vi "Tcheck.vi"(0 "TargetT":dbl, 1 "timeout (s)":dbl=600.0, 2 "Direct reading":bool, 3 "VI name":string="Tmonitor.vi", 5 "target T\nDT error":dbl=0.001 format="%#_13g", 7 "VISA resource name":refnum<visa-resource-name>, 9 "T to watch":string="T0", 11 "T control mode":u16(ring) items=["Tprobe", "Tsorb", "Fast Tsweep", "Skip T stable"], 14 "Pass":bool) -> (4 "Temp OK":bool, 6 "Temp close to\nTarget T":bool, 10 "time passed (s)":dbl=37.23 format="%#_4g", 15 "Temp":dbl=155.435 format="%#_4g")   [LabVIEW 2025]
uses:
  <vilib>/Analysis/baseanly.llb/Mean (DBL).vi
  <vilib>/Analysis/NI_AALBase.lvlib
panel:
  in  "Controller":u16(ring) items=["LS370", "LS340", "LS336"]
  in  "Channel":u16(ring) items=["A", "B", "C", "D", "4"]
  out "meanT":dbl format="%0.2f"
  out "min T":dbl
  out "max T":dbl
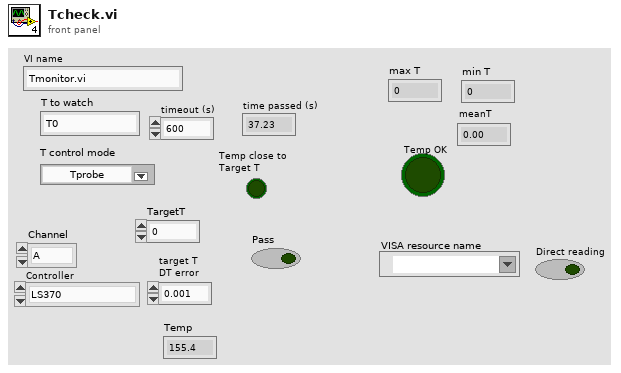
[diagram p1: front panel]
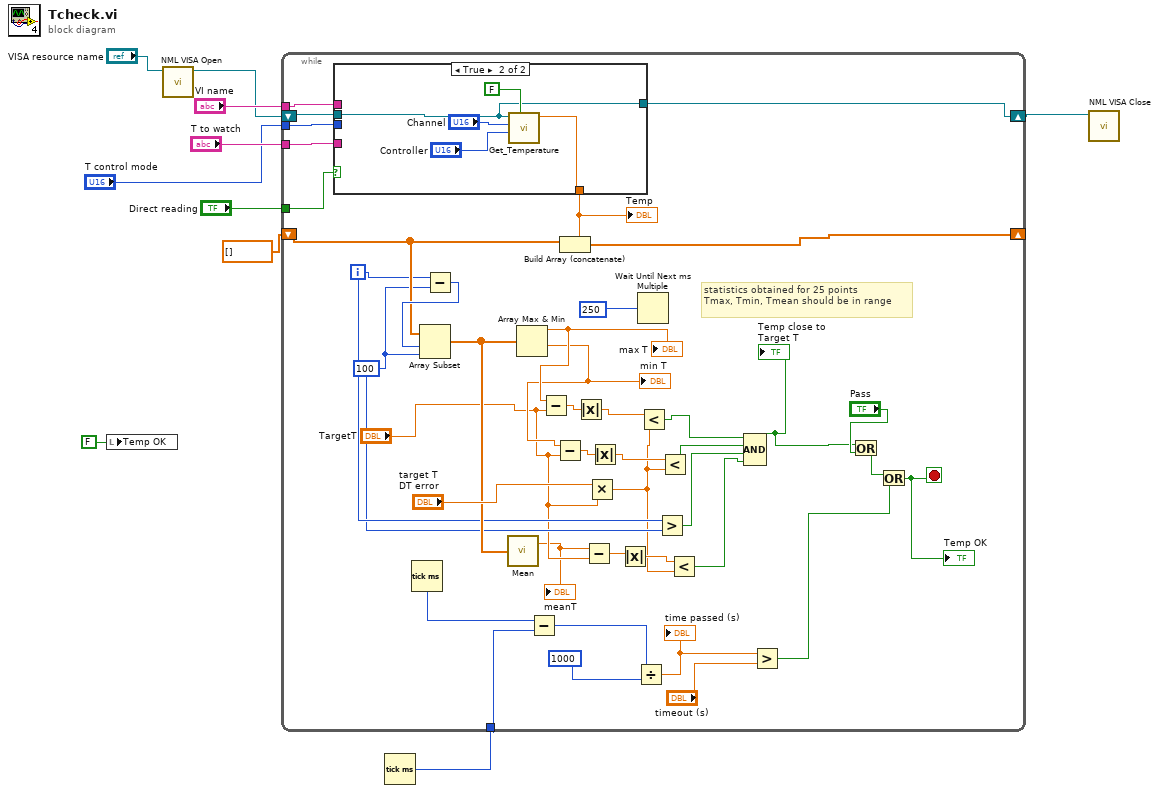
[diagram p0: block diagram]
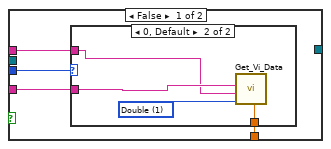
[diagram p2: hidden frame]
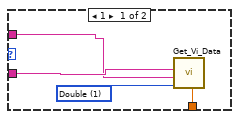
[diagram p3: hidden frame]
diagram:
  n1 = local write "Temp OK"(FALSE ("Temp OK")) -> ()
  n2 = call "NML VISA Open.vi"("VISA resource name"="VISA resource name") -> ("VISA resource name out"=w2:refnum<visa-resource-name>)  [unwired: 9 in, 1 out]
  n3 = Tick Count (ms)() -> (millisecond timer value=w10:u32)
  n4 = while {
    tunnel: w10 -> [w40]
    shift-right: [w37] -> _
    shift-left: dbl[] [] -> [w35]
    tunnel: "T to watch" -> [w17]
    tunnel: "T control mode" -> [w16]
    tunnel: "VI name" -> [w15]
    tunnel: "Direct reading" -> [w13]
    shift-right: [w11] -> w1
    shift-left: w2 -> [w12]
    i -> [w29]
    stop <- w14 stop-if-true
    w28 = 100 ("length")
    # "statistics obtained for 25 points\nTmax, Tmin, Tmean should be in range"
    n5 = case shown="True" w13 {
      tunnel: [w55 w65] -> w38
      tunnel: w17 -> [w54 _]
      tunnel: w16 -> [w53 _]
      tunnel: w15 -> [w52 _]
      tunnel: w12 -> [_ w64]
      tunnel: [_ w64] -> w11
      frame False {
        n6 = case shown="0, Default" w53 {
          tunnel: [w58 w62] -> w55
          tunnel: w54 -> [w57 w61]
          tunnel: w52 -> [w56 w60]
          frame 1 {
            w59 = u16 1 items=["String", "Double", "Boolean", "Variant"] ("Data Type")
            n7 = call "Get_Vi_Data.vi"("Data Type"=w59, "VI name"=w56, "Control Name"=w57) -> ("Data (Double)"=w58:dbl)  [unwired: 4 in, 4 out]
          }
          frame 0, Default {
            w63 = u16 1 items=["String", "Double", "Boolean", "Variant"] ("Data Type")
            n8 = call "Get_Vi_Data.vi"("Data Type"=w63, "VI name"=w60, "Control Name"=w61) -> ("Data (Double)"=w62:dbl)  [unwired: 4 in, 4 out]
          }
        }
      }
      frame True {
        n9 = call "Get_Temperature.vi"("Res?"=FALSE, "Controller"="Controller", "Channel"="Channel", "VISA resource name"=w64) -> ("Temperature"=w65:dbl)  [unwired: 6 in, 1 out]
      }
    }
    "Temp" <- w38
    n10 = Tick Count (ms)() -> (millisecond timer value=w47:u32)
    n11 = Subtract(x=w29, y=w28) -> (x-y=w36:i32)
    n12 = Array Subset(array=w35, index=w36, length=w28) -> (w30:dbl[])
    n13 = call-poly <vilib>:"Mean.vi"("X"=w30) -> ("mean"=w23:dbl)  [unwired: 1 out]
    "meanT" <- w23
    n14 = Array Max & Min(array=w30) -> (max value=w34:dbl, min value=w31:dbl)  [unwired: 2 out]
    "max T" <- w34
    "min T" <- w31
    n15 = Subtract(x=w47, y=w40) -> (x-y=w46:u32)
    n16 = Subtract(x=w34, y="TargetT") -> (x-y=w49:dbl)
    n17 = Subtract(x=w31, y="TargetT") -> (x-y=w32:dbl)
    n18 = Build Array (concatenate)(w35, w38) -> (w37:dbl[])
    n19 = Absolute Value(x=w49) -> (abs(x)=w50:dbl)
    n20 = Subtract(x=w23, y="TargetT") -> (x-y=w21:dbl)
    n21 = Multiply(x="target T\nDT error", y="TargetT") -> (x*y=w20:dbl)
    n22 = Absolute Value(x=w32) -> (abs(x)=w33:dbl)
    n23 = Absolute Value(x=w21) -> (abs(x)=w22:dbl)
    n24 = Divide(x=w46, y=u32 1000) -> (x/y=w44:dbl)
    "time passed (s)" <- w44
    n25 = Wait Until Next ms Multiple(millisecond multiple=u32 250 ("200")) -> ()  [unwired: 1 out]
    n26 = Less?(x=w50, y=w20) -> (x < y?=w27:bool)
    n27 = Greater?(x=w29, y=w28) -> (0:w25:bool)
    n28 = Less?(x=w33, y=w20) -> (x < y?=w26:bool)
    n29 = Less?(x=w22, y=w20) -> (x < y?=w19:bool)
    n30 = Compound Arithmetic op=AND(w27, w26, w25, w19) -> (w18:bool)
    "Temp close to\nTarget T" <- w18
    n31 = Greater?(x=w44, y="timeout (s)") -> (0:w41:bool)
    n32 = Or(x=w18, y="Pass") -> (x .or. y?=w42:bool)
    n33 = Or(x=w42, y=w41) -> (x .or. y?=w14:bool)
    "Temp OK" <- w14
  }
  n34 = call "NML VISA Close.vi"("VISA resource name"=w1) -> ()  [unwired: 10 in, 1 out]
